vi "Run_Core.vi"(0 "Message Popup in":refnum<class "DMM.lvclass">, 11 "error in (no error)":errorcluster) -> (4 "Message Popup out":refnum<class "DMM.lvclass">, 6 "Return":variant, 15 "error out":errorcluster)   [LabVIEW 2016, in "DMM.lvclass"]
uses:
  DMM.lvclass
  DMM.lvclass/DMM.ctl
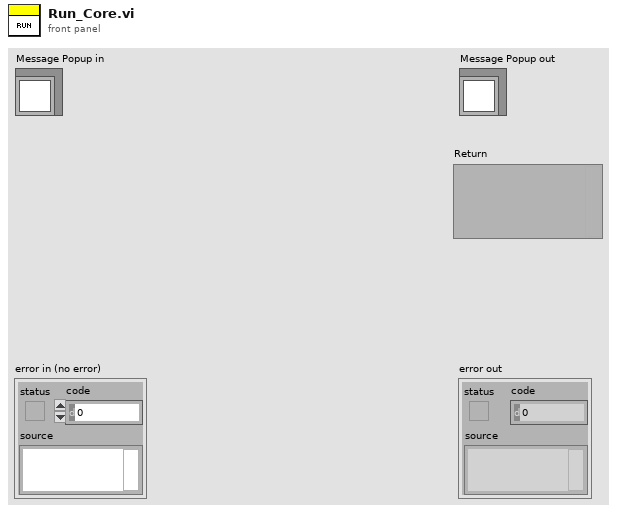
[diagram p1: front panel]
types:
  T1 = typedef "DMM.lvclass/Function List.ctl" = enum16{"init", "measure", "close", "close all"}
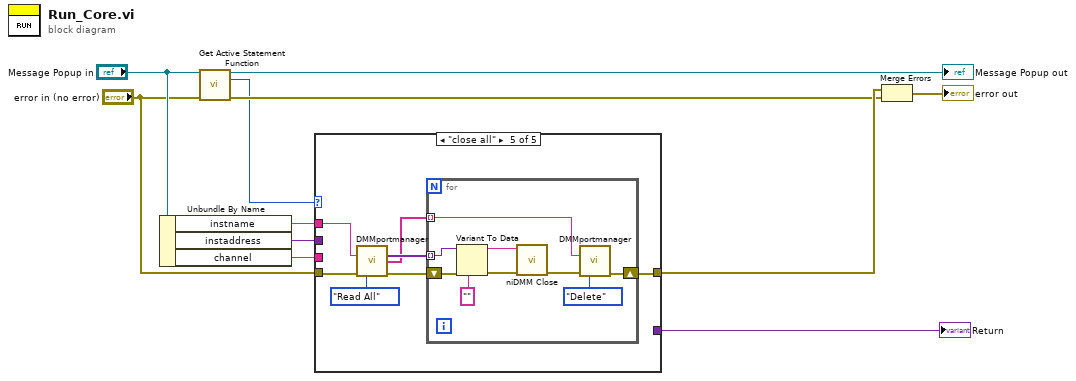
[diagram p0: block diagram]
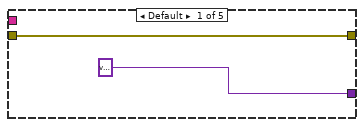
[diagram p2: hidden frame]
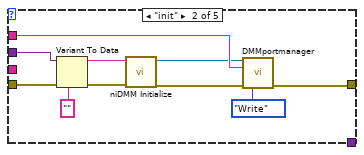
[diagram p3: hidden frame]
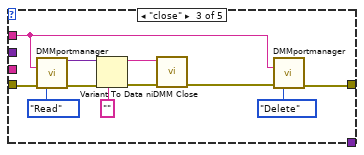
[diagram p4: hidden frame]
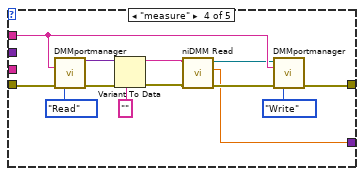
[diagram p5: hidden frame]
diagram:
  n1 = Unbundle By Name("Message Popup in") -> ("instname"=w1:string, "instaddress"=w7:variant, "channel"=w8:string)
  n2 = call "Get Active Statement Function.vi"("Statement in"="Message Popup in", "error in (no error)"="error in (no error)") -> ("Statement out"=→"Message Popup out":refnum<class "DMM.lvclass">, "Function List"=w3:T1, "error out"=w5:errorcluster)  [unwired: 11 in]
  n3 = case shown="\"close all\"" w3 {
    tunnel: "error in (no error)" -> [w13 w22 w26 w42 w51]
    tunnel: w8 -> [_ _ _ _ _]
    tunnel: w7 -> [_ w23 _ _ _]
    tunnel: [w13 w15 w32 w45 w54] -> w6
    tunnel: [variant ("lefttocomma") _ _ w35 _] -> w2
    tunnel: w1 -> [_ w18 w25 w41 w50]
    frame Default {
    }
    frame "init" {
      n4 = Variant To Data(error in=w22, type="", Variant=w23) -> (data=w19:string, error out=w21:errorcluster)
      n5 = call <instrlib>:"niDMM Initialize.vi"("error in (no error)"=w21, "Instrument Descriptor"=w19) -> ("error out"=w17:errorcluster, "instrument handle out"=w16:refnum<k15>)  [unwired: 8 in]
      n6 = call "DMMportmanager.vi"("port in"=w16, "Name"=w18, "error in (no error)"=w17, "Action"=enum16{"Read", "Write", "Read All", "Delete"}."Write") -> ("error out"=w15:errorcluster)  [unwired: 8 in, 3 out]
    }
    frame "close" {
      n7 = call "DMMportmanager.vi"("Name"=w25, "error in (no error)"=w26, "Action"=enum16{"Read", "Write", "Read All", "Delete"}."Read") -> ("port"=w24:variant, "error out"=w28:errorcluster)  [unwired: 9 in, 2 out]
      n8 = Variant To Data(error in=w28, type="", Variant=w24) -> (data=w31:string, error out=w30:errorcluster)
      n9 = call <instrlib>:"niDMM Close.vi"("error in (no error)"=w30, "instrument handle"=w31) -> ("error out"=w29:errorcluster)  [unwired: 9 in]
      n10 = call "DMMportmanager.vi"("Name"=w25, "error in (no error)"=w29, "Action"=enum16{"Read", "Write", "Read All", "Delete"}."Delete") -> ("error out"=w32:errorcluster)  [unwired: 9 in, 3 out]
    }
    frame "measure" {
      n11 = call "DMMportmanager.vi"("Name"=w41, "error in (no error)"=w42, "Action"=enum16{"Read", "Write", "Read All", "Delete"}."Read") -> ("port"=w40:variant, "error out"=w44:errorcluster)  [unwired: 9 in, 2 out]
      n12 = Variant To Data(error in=w44, type="", Variant=w40) -> (data=w39:string, error out=w38:errorcluster)
      n13 = call <instrlib>:"niDMM Read.vi"("error in (no error)"=w38, "instrument handle"=w39) -> ("error out"=w37:errorcluster, "Measurement"=w35:dbl, "instrument handle out"=w36:refnum<k15>)  [unwired: 7 in]
      n14 = call "DMMportmanager.vi"("port in"=w36, "Name"=w41, "error in (no error)"=w37, "Action"=enum16{"Read", "Write", "Read All", "Delete"}."Write") -> ("error out"=w45:errorcluster)  [unwired: 8 in, 3 out]
    }
    frame "close all" {
      n15 = call "DMMportmanager.vi"("Name"=w50, "error in (no error)"=w51, "Action"=enum16{"Read", "Write", "Read All", "Delete"}."Read All") -> ("port[]"=w49:variant[], "port names[]"=w48:string[], "error out"=w53:errorcluster)  [unwired: 9 in, 1 out]
      n16 = for {
        shift-right: [w61] -> w54
        shift-left: w53 -> [w57]
        tunnel: w49 -> [w56] mode=indexing
        tunnel: w48 -> [w55] mode=indexing
        n17 = Variant To Data(error in=w57, type="", Variant=w56) -> (data=w60:string, error out=w59:errorcluster)
        n18 = call <instrlib>:"niDMM Close.vi"("error in (no error)"=w59, "instrument handle"=w60) -> ("error out"=w58:errorcluster)  [unwired: 9 in]
        n19 = call "DMMportmanager.vi"("Name"=w55, "error in (no error)"=w58, "Action"=enum16{"Read", "Write", "Read All", "Delete"}."Delete") -> ("error out"=w61:errorcluster)  [unwired: 9 in, 3 out]
      }
    }
  }
  "Return" <- w2
  n20 = Merge Errors(w6, w5) -> (→"error out":errorcluster)
